vi "Nicholas IO Server.vi"() -> ()   [LabVIEW 2015]
uses:
  RS485 In.ctl
  Serial Data In.ctl
  PAS Modulation.ctl
  <vilib>/rvi/eio/common/nirviEmuClasses.ctl
  Port.ctl
  <vilib>/Platform/TimedLoop/XDataNode/timing_clust.ctl
  <vilib>/Platform/TimedLoop/XDataNode/nitl_modes.ctl
  <vilib>/Platform/TimedLoop/XDataNode/wakeup.ctl
  <vilib>/rvi/FXPMathLib/basic elements/FxpIntAccumulator/subVIs/nifxpmath_IntAccumulator_SimConfig.ctl
  <vilib>/rvi/Emulation/niFpgaSctlEmulationGetInTimedLoop.vi
  <vilib>/rvi/Emulation/niFpgaProcessEmulError.vi
  <vilib>/rvi/eio/common/nirviEmuTemplateMethod_errors.vi
  <vilib>/rvi/Emulation/niFpgaEmulationIsFPGAContextNoSignature.vi
  <vilib>/rvi/DataTransferAndStorage/Container/Common/niFpgaContainerGetUniqueNameForEmu.vi
  <vilib>/rvi/Memory/Memory_Emulation/niFpgaMemoryEmulationCacheClearOnFirstRun.vi
  <vilib>/rvi/Memory/Memory_Emulation/nirvimemoryEmulationManagerCache_MakeExclusive.vi
  <vilib>/rvi/Memory/Memory_Emulation/niFpgaMemoryEmulationValidateCache.vi
  <vilib>/rvi/Memory/Memory_Emulation/nirvimemoryEmulationManagerCache_InsertValue.vi
  <vilib>/Utility/error.llb/Clear Errors.vi
  <vilib>/rvi/Memory/Memory_Emulation/nirvimemoryEmulationManagerCache_ReleaseExclusive.vi
  <vilib>/rvi/Memory/Memory_Emulation/nirvimemoryEmulationManagerCache_GetValue.vi
  <vilib>/rvi/Memory/Memory_Emulation/nirvimemoryEmulationManagerCache_SetValue.vi
  <vilib>/rvi/Emulation/niFpgaGetClockAttributes.vi
  <vilib>/rvi/Emulation/niFpgaEmulationReportErrorSimple.vi
  <vilib>/rvi/Emulation/niFpgaCriticalErrorInLSC.vi
  <vilib>/rvi/FXPMathLib/basic elements/FxpIntAccumulator/simVIs/DllFxpIntAccumulator_sub.vi
  <vilib>/eio/EIOGrowableMethodNode/genericMethod/EIOGrowableMethodNode.xnode
  <vilib>/rvi/eio/nirviEIOMethodImplementation/nirviEIOMethodImplementation.xnode
  <vilib>/rvi/eio/nirviErrorMerge/nirviErrorMerge.xnode
  <vilib>/rvi/DataTransferAndStorage/Container/XNode/niFpgaContainer.xnode
  <vilib>/rvi/DataTransferAndStorage/Register/Emulation/niFpgaRegisterEmulation.vi
  <vilib>/Platform/TimedLoop/XDataNode/XDataNode.xnode
  <vilib>/eio/EIONode/EIONode.xnode
  <vilib>/rvi/FXPMathLib/basic elements/FxpIntAccumulator/XNode/nifxpmath_IntAccumulator.xnode
  <vilib>/rvi/FXPMathLib/basic elements/FxpDiscreteDelay/XNode/nifxpmath_DiscreteDelay.xnode
  <vilib>/rvi/FXPMathLib/FxpMul/XNode/nifxpmath_Multiplier.xnode
  <vilib>/Platform/TimedLoop/XDataNode/XDNodeRunTimeDep.lvlib
  <vilib>/rvi/FXPMathLib/sim/FxpSim.dll
panel:
  out "DI Out":u8
  out "DO Out":u16
  in  "DO In":u16
  out "Version":i64=3288624
  in  "pDC":fxp<+,32,0>
  in  "Wave":T1 {"Mod" items=["Sine", "Square"]}
  out "Port4 Out":T2
  in  "Port4 In":T3={"Data"=[0, 0, 0, 0, 0, 0, 0, 0, 0, 0, 0, 0, 0, 0, 0, 0, 0, 0, 0, 0], "NumBytes"=0, "RS485_Cmd"=enum."Idle", "Timeout (ms)"=0}
  out "Port3 Out":T2
  in  "Port3 In":T3={"Data"=[0, 0, 0, 0, 0, 0, 0, 0, 0, 0, 0, 0, 0, 0, 0, 0, 0, 0, 0, 0], "NumBytes"=0, "RS485_Cmd"=enum."Idle", "Timeout (ms)"=0}
  out "Port2 Out":T2
  in  "Port2 In":T3={"Data"=[0, 0, 0, 0, 0, 0, 0, 0, 0, 0, 0, 0, 0, 0, 0, 0, 0, 0, 0, 0], "NumBytes"=0, "RS485_Cmd"=enum."Idle", "Timeout (ms)"=0}
  in  "Port1 In":T3={"Data"=[0, 0, 0, 0, 0, 0, 0, 0, 0, 0, 0, 0, 0, 0, 0, 0, 0, 0, 0, 0], "NumBytes"=0, "RS485_Cmd"=enum."Idle", "Timeout (ms)"=0}
  out "Port1 Out":T2
  in  "Transmit?":bool
  in  "CRDSampData":u32
  in  "Speaker":cluster{"Vscale":fxp<+,32,0>, "Offset":i16}
  in  "Stop":bool
  out "HK Data":fxp<+/-,16,5>[](array[numeric])
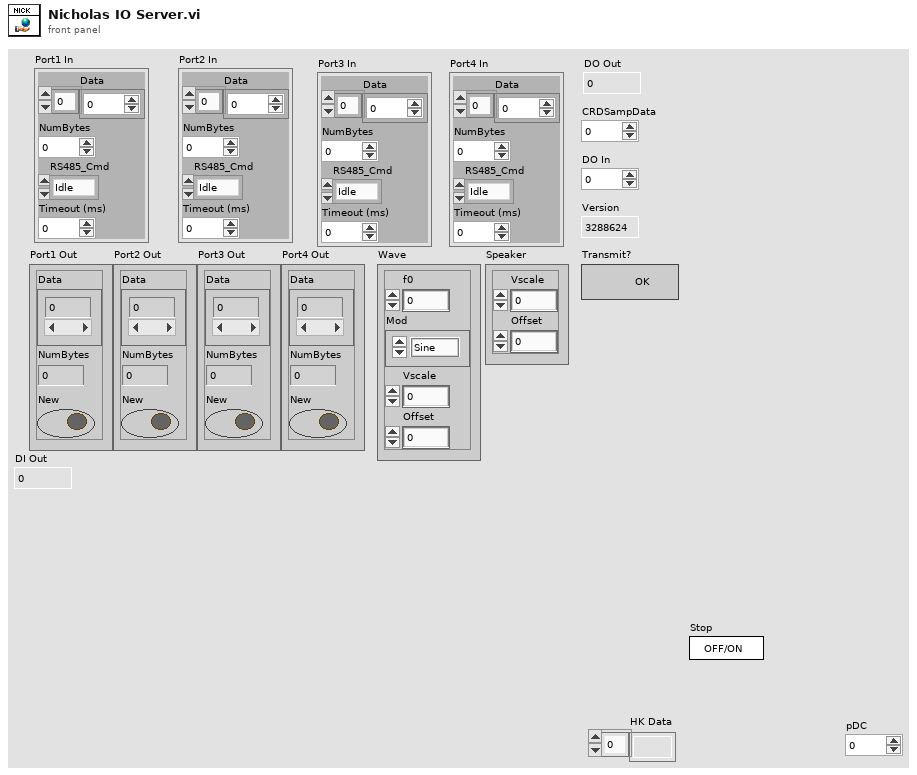
[diagram p1: front panel]
types:
  T1 = typedef "PAS Modulation.ctl" = cluster{"f0":fxp<+,32,0>, "Mod":u8, "Vscale":fxp<+,32,0>, "Offset":i16}
  T2 = typedef "RS485 In.ctl" = cluster{"Data":u8[], "NumBytes":i32, "New":bool}
  T3 = typedef "Serial Data In.ctl" = cluster{"Data":u8[], "NumBytes":i32, "RS485_Cmd":enum8{"Read", "Write", "Idle"}, "Timeout (ms)":i32}
  T4 = typedef "nirviEmuClasses.ctl" = enum16{"IO Read", "IO Write", "Method", "Property Read", "Property Write"}
  T5 = typedef "Port.ctl" = enum8{"Port 1", "Port 2", "Port 3", "Port 4", "None"}
  T6 = typedef "XDNodeRunTimeDep.lvlib/timing_clust.ctl" = cluster{"Expected End [f-1]":u64, "Actual End [f-1]":u64, "Finished Late? [f-1]":bool, "Expected End [i-1]":u64, "Actual End [i-1]":u64, "Finished Late? [i-1]":bool, "Expected Start [i]":u64, "Actual Start [i]":u64, "Expected Start [f]":u64, "Actual Start [f]":u64, "Source Name":string, "Structure Name":string, "Period":i64, "Deadline":i64, "Offset":i64, "Start":i64, "Priority":i32, "Timeout":i32, "Mode":T7, "Wakeup Reason":T8, "Error":errorcluster, "Source Type":string, "Secondary Source Type":string, "Global End Time":u64, "Global Start Time":u64, "Frame Duration":u64, "Iteration Duration":u64, "Assigned CPU":i32, "I/O Scan Engine Mode":u32}
  T7 = typedef "XDNodeRunTimeDep.lvlib/nitl_modes.ctl" = enum32{"No Change", "Process missed periods, maintain original phase", "Discard missed periods, maintain original phase", "Process missed periods, ignore original phase", "Discard missed periods, ignore original phase"}
  T8 = typedef "XDNodeRunTimeDep.lvlib/wakeup.ctl" = enum32{"Normal", "Aborted", "Asynchronous wakeup", "Timing source error", "Timed loop error", "Timeout"}
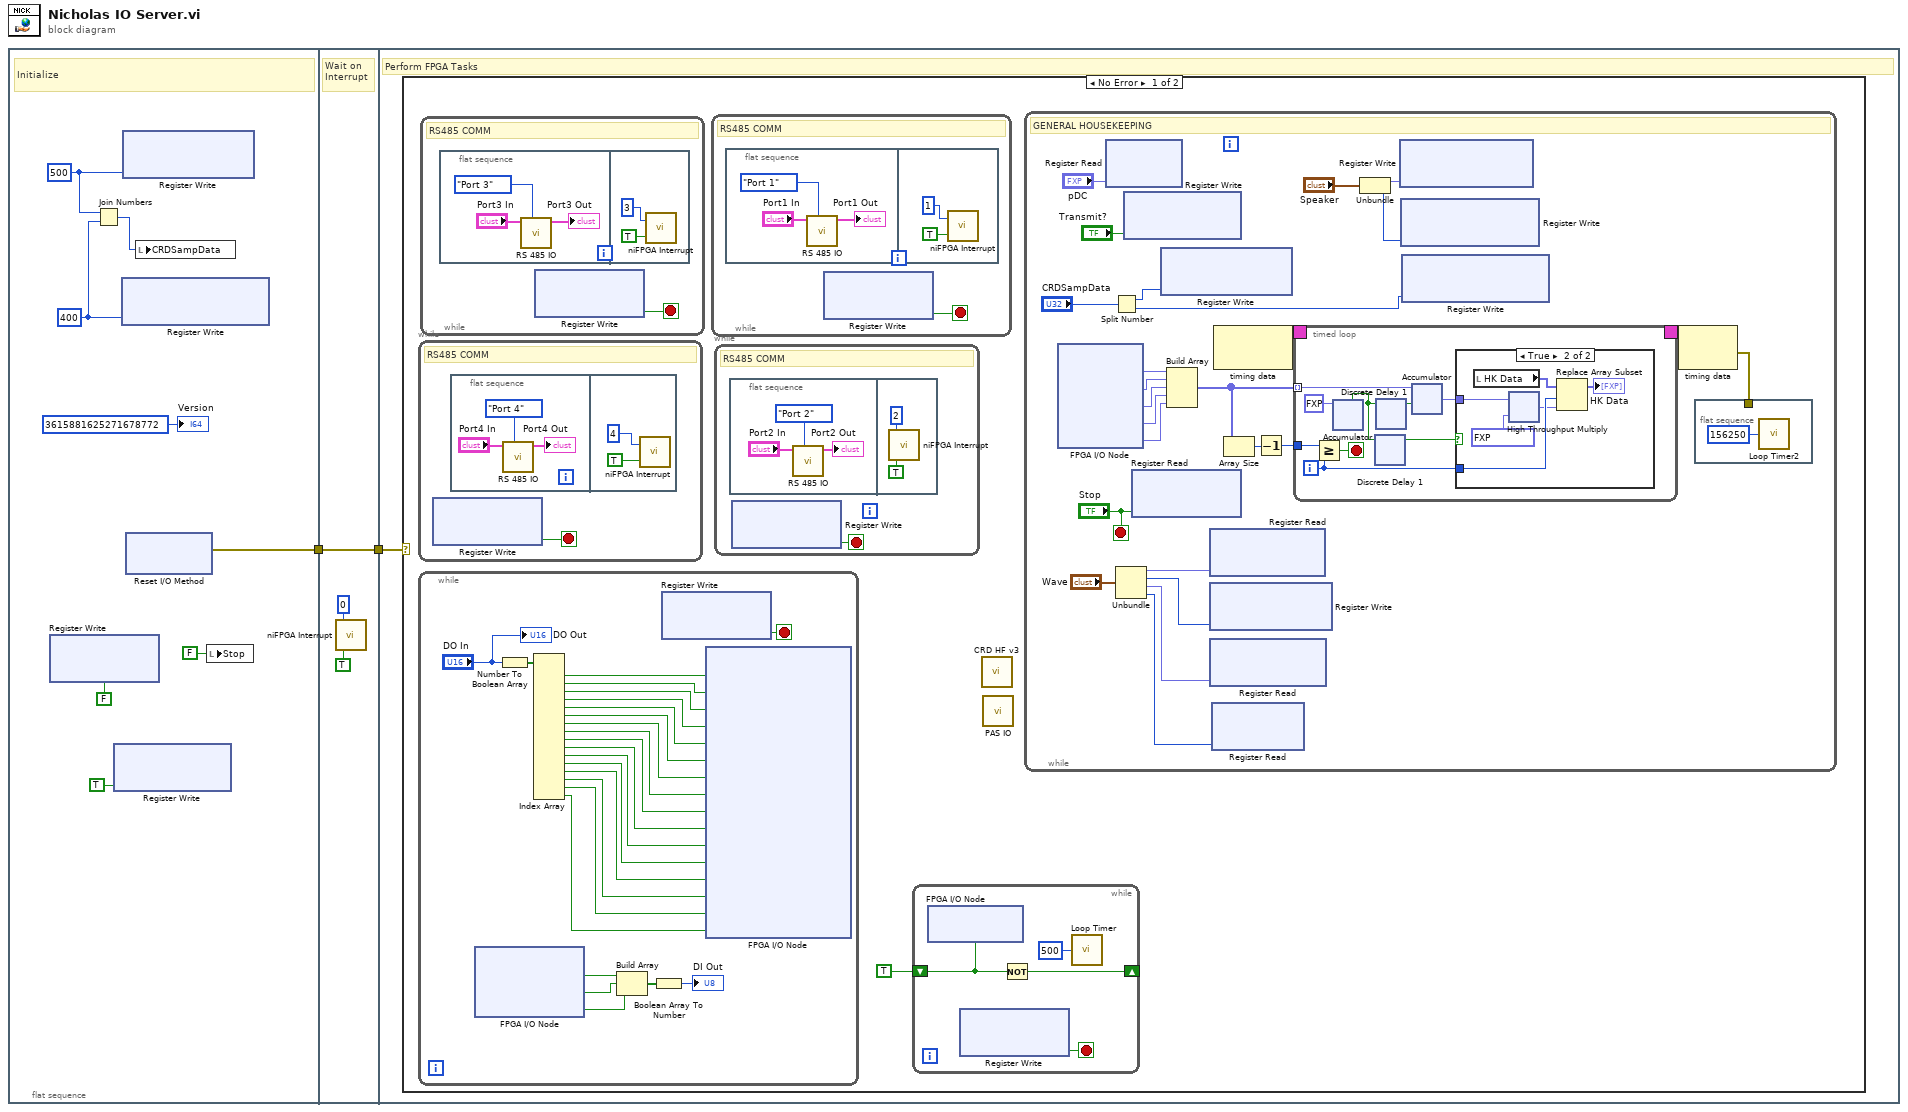
[diagram p0: block diagram]
diagram:
  n1 = flat-sequence {
    tunnel: [w10] -> w2
    tunnel: w2 -> [w57]
    tunnel: [w57] -> w1
    tunnel: w1 -> [w58]
    frame #0 {
      w5 = u16 500 ("Data")
      w4 = u16 400 ("Data")
      # "Initialize"
      n2 = xnode ("Register Write")("Data"=FALSE) -> ()  [unwired: 1 in, 1 out]
      n3 = Join Numbers(hi=w5, lo=w4) -> ((hi.lo)=w3:u32)
      n4 = xnode ("Register Write")("Data"=TRUE) -> ()  [unwired: 1 in, 1 out]
      n5 = xnode ("Register Write")("Data"=w4) -> ()  [unwired: 1 in, 1 out]
      n6 = xnode ("Register Write")("Data"=w5) -> ()  [unwired: 1 in, 1 out]
      n7 = xnode "Reset I/O Method"() -> ("error out"=w10:errorcluster)  [unwired: 2 in, 1 out]
      n8 = local write "CRDSampData"(w3) -> ()
      n9 = local write "Stop"(FALSE ("Stop")) -> ()
      "Version" <- i64 3615881625271678772 ("Data")
    }
    frame #1 {
      # "Wait on Interrupt"
      n10 = call <vilib>:"niFPGA Interrupt.vi"("Wait Until Cleared (F)"=TRUE ("Wait Until Cleared"), "IRQ Number (0)"=u8 0 ("IRQ Number")) -> ()  [unwired: 1 in]
    }
    frame #2 {
      # "Perform FPGA Tasks"
      n11 = case shown="No Error" w58 {
        frame No Error {
          n12 = while {
            stop <- w70 stop-if-true
            # "RS485 COMM"
            n13 = xnode ("Register Write")() -> ("Data"=w70:bool)  [unwired: 1 in, 1 out]
            n14 = flat-sequence {
              frame #0 {
                n15 = call "RS 485 IO.vi"("Port"=Port."Port 4", "Input in"="Port4 In") -> ("Input out"=→"Port4 Out":T2)  [unwired: 8 in]
              }
              frame #1 {
                n16 = call <vilib>:"niFPGA Interrupt.vi"("Wait Until Cleared (F)"=TRUE, "IRQ Number (0)"=u8 4) -> ()  [unwired: 1 in]
              }
            }
          }
          n17 = while {
            stop <- w111 stop-if-true
            n18 = xnode "FPGA I/O Node"() -> ("hb 1 status 1"=w92:bool, "hb 1 status 2"=w91:bool, "Interlock"=w90:bool)  [unwired: 3 in, 3 out]
            n19 = Number To Boolean Array(number="DO In") -> (Boolean array=w109:bool[])
            n20 = Index Array(array=w109) -> (element #1=w108:bool, element #2=w107:bool, element #3=w106:bool, element #4=w105:bool, element #5=w104:bool, element #6=w103:bool, element #7=w102:bool, element #8=w101:bool, element #9=w100:bool, element #10=w99:bool, element #11=w98:bool, element #12=w97:bool, element #13=w96:bool, element #14=w95:bool, element #15=w94:bool, element #16=w93:bool)  [unwired: 16 in]
            n21 = Build Array(w92, w91, w90) -> (w89:bool[])
            n22 = Boolean Array To Number(Boolean array=w89) -> (number=→"DI Out":u8)
            n23 = xnode ("Register Write")() -> ("Data"=w111:bool)  [unwired: 1 in, 1 out]
            n24 = xnode "FPGA I/O Node"("uv light ctl 1"=w108, "uv light ctl 2"=w107, "uv light enable"=w106, "Laser Enable"=w105, "PAS Speaker"=w104, "Compressor Enable"=w103, "Vacuum Pump"=w102, "O3 Add"=w101, "Scrubber Test"=w100, "Pressure Meas 1"=w99, "Pressure Meas 2"=w98, "hb 1 ctl 1"=w97, "hb 1 ctl 2"=w96, "CRD Laser Enable"=w95, "PMT Enable"=w94, "Fan Enable"=w93) -> ()  [unwired: 16 in, 16 out]
            "DO Out" <- "DO In"
          }
          n25 = while {
            stop <- w76 stop-if-true
            # "RS485 COMM"
            n26 = flat-sequence {
              frame #0 {
                n27 = call "RS 485 IO.vi"("Port"=Port."Port 3", "Input in"="Port3 In") -> ("Input out"=→"Port3 Out":T2)  [unwired: 8 in]
              }
              frame #1 {
                n28 = call <vilib>:"niFPGA Interrupt.vi"("Wait Until Cleared (F)"=TRUE, "IRQ Number (0)"=u8 3) -> ()  [unwired: 1 in]
              }
            }
            n29 = xnode ("Register Write")() -> ("Data"=w76:bool)  [unwired: 1 in, 1 out]
          }
          n30 = while {
            stop <- w82 stop-if-true
            # "RS485 COMM"
            n31 = flat-sequence {
              frame #0 {
                n32 = call "RS 485 IO.vi"("Port"=Port."Port 1", "Input in"="Port1 In") -> ("Input out"=→"Port1 Out":T2)  [unwired: 8 in]
              }
              frame #1 {
                n33 = call <vilib>:"niFPGA Interrupt.vi"("Wait Until Cleared (F)"=TRUE, "IRQ Number (0)"=u8 1) -> ()  [unwired: 1 in]
              }
            }
            n34 = xnode ("Register Write")() -> ("Data"=w82:bool)  [unwired: 1 in, 1 out]
          }
          n35 = while {
            stop <- w64 stop-if-true
            # "RS485 COMM"
            n36 = flat-sequence {
              frame #0 {
                n37 = call "RS 485 IO.vi"("Port"=Port."Port 2", "Input in"="Port2 In") -> ("Input out"=→"Port2 Out":T2)  [unwired: 8 in]
              }
              frame #1 {
                n38 = call <vilib>:"niFPGA Interrupt.vi"("Wait Until Cleared (F)"=TRUE, "IRQ Number (0)"=u8 2) -> ()  [unwired: 1 in]
              }
            }
            n39 = xnode ("Register Write")() -> ("Data"=w64:bool)  [unwired: 1 in, 1 out]
          }
          n40 = while {
            shift-right: [w61] -> _
            shift-left: TRUE -> [w62]
            stop <- w60 stop-if-true
            n41 = xnode "FPGA I/O Node"("Heartbeat"=w62) -> ()  [unwired: 1 in, 1 out]
            n42 = xnode ("Register Write")() -> ("Data"=w60:bool)  [unwired: 1 in, 1 out]
            n43 = Not(x=w62) -> (.not. x?=w61:bool)
            n44 = call "Loop Timer"("Count(mSec)"=u32 500 ("Count(Ticks)")) -> ()  [unwired: 1 out]
          }
          n45 = call "CRD HF v3.vi"() -> ()  [unwired: 12 in]
          n46 = call "PAS IO.vi"() -> ()  [unwired: 20 in]
          n47 = while {
            stop <- "Stop" stop-if-true
            # "GENERAL HOUSEKEEPING"
            n48 = xnode "FPGA I/O Node"() -> ("Tcomp"=w130:fxp<+/-,26,5>, "TEC hot"=w131:fxp<+/-,26,5>, "Troom"=w132:fxp<+/-,26,5>, "Box"=w133:fxp<+/-,26,5>, "Cell"=w134:fxp<+/-,26,5>)  [unwired: 5 in, 5 out]
            n49 = xnode ("Register Read")("Data"="pDC") -> ()  [unwired: 1 in, 1 out]
            n50 = Split Number(x="CRDSampData") -> (hi(x)=w113:u16, lo(x)=w112:u16)
            n51 = Unbundle("Wave") -> ("f0"=w120:fxp<+,32,0>, "Mod"=w115:u8, "Vscale"=w118:fxp<+,32,0>, "Offset"=w119:i16)
            n52 = xnode ("Register Write")("Data"="Transmit?") -> ()  [unwired: 1 in, 1 out]
            n53 = xnode ("Register Read")("Data"="Stop") -> ()  [unwired: 1 in, 1 out]
            n54 = xnode ("Register Write")("Data"=w113) -> ()  [unwired: 1 in, 1 out]
            n55 = Build Array(w130, w131, w132, w133, w134) -> (w129:fxp<+/-,26,5>[])
            n56 = xnode ("Register Read")("Data"=w120) -> ()  [unwired: 1 in, 1 out]
            n57 = xnode ("Register Write")("Data"=w115) -> ()  [unwired: 1 in, 1 out]
            n58 = xnode ("Register Read")("Data"=w118) -> ()  [unwired: 1 in, 1 out]
            n59 = xnode ("Register Read")("Data"=w119) -> ()  [unwired: 1 in, 1 out]
            n60 = node-c288() -> (w136:T6)  [unwired: 1 in]
            n61 = Array Size(array=w129) -> (size(s)=w128:i32)
            n62 = Decrement(x=w128) -> (x-1=w127:i32)
            n63 = timed-loop {
              timing: w136 -> [_]
              timing-out: [_] -> w135
              tunnel: w129 -> [w144] mode=indexing
              tunnel: w127 -> [w146]
              i -> [w138]
              stop <- w145 stop-if-true
              n64 = Greater Or Equal?(x=w146, y=w138) -> (x >= y?=w145:bool)
              n65 = xnode "Accumulator"("x"=fxp<+,1,1> 1.0) -> ("carry-out/inverted borrow-out"=w141:bool)  [unwired: 4 in, 1 out]
              n66 = xnode ("Discrete Delay 1")("D"=w141) -> ("Q"=w140:bool)
              n67 = xnode ("Discrete Delay 1")("D"=w141) -> ("Q"=w142:bool)
              n68 = xnode "Accumulator"("x"=w144, "load (F)"=w142) -> ("s"=w139:fxp<+/-,32,11>)  [unwired: 3 in, 1 out]
              n69 = case shown="True" w140 {
                tunnel: w139 -> [_ w152]
                tunnel: w138 -> [_ w150]
                frame False {
                }
                frame True {
                  n70 = local read "HK Data"() -> (w151:fxp<+/-,16,5>[])
                  n71 = xnode ("High Throughput Multiply")("x"=w152, "y"=fxp<+,32,1> 0.00390625) -> ("x*y"=w149:fxp<+/-,16,5>)
                  n72 = Replace Array Subset(array=w151, new element=w149, index=w150) -> (→"HK Data":fxp<+/-,16,5>[])
                }
              }
            }
            n73 = Unbundle("Speaker") -> ("Vscale"=w116:fxp<+,32,0>, "Offset"=w122:i16)
            n74 = xnode ("Register Write")("Data"=w116) -> ()  [unwired: 1 in, 1 out]
            n75 = xnode ("Register Write")("Data"=w122) -> ()  [unwired: 1 in, 1 out]
            n76 = xnode ("Register Write")("Data"=w112) -> ()  [unwired: 1 in, 1 out]
            n77 = node-c288(w135) -> (w126:errorcluster)
            n78 = flat-sequence {
              tunnel: w126 -> [_]
              frame #0 {
                n79 = call "Loop Timer2"("Count(Ticks)"=u32 156250 ("Count(mSec)")) -> ()  [unwired: 1 out]
              }
            }
          }
        }
        frame Error {
        }
      }
    }
  }
